vi "Try 1.vi"() -> ()   [LabVIEW 2014]
panel:
  out "String":string
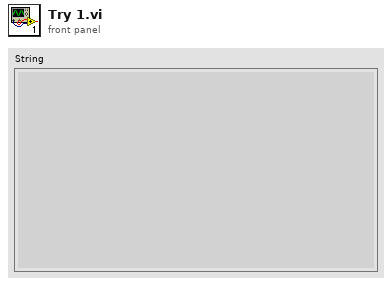
[diagram p1: front panel]
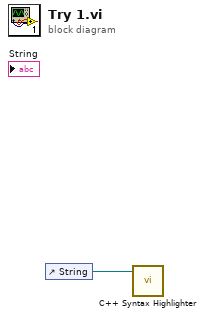
[diagram p0: block diagram]
diagram:
  n1 = control-ref of="String"() -> (w1:refnum<vi>)
  n2 = call "C++ Syntax Highlighter.vi"("control/indicator refnum in"=w1) -> ()  [unwired: 10 in, 1 out]
